vi "Get SMO Database Paths.vi"(5 "getAll Cluster":variant, 7 "Paths":string="llab_038:d000(TEST_TABLE--Temperature(Kelvin))\nllab_038:d002(TEST_TABLE--voltage 2(volts))\nllab_038:b000(TEST_TABLE--ON?())\nllab_038:v001(TEST_TABLE--sample())", 8 "error in (no error)":errorcluster, 11 "Instrument.AFM_DLog in":refnum<class "Instrument.AFM_DLog.lvclass">) -> (0 "error out":errorcluster, 2 "Paths":string, 3 "Instrument.AFM_DLog out":refnum<class "Instrument.AFM_DLog.lvclass">)   [LabVIEW 2019, in "Instrument.AFM_DLog.lvclass"]
uses:
  Instrument.AFM_DLog.lvclass
  Typedefs/Instrument.AFM_DLog.getAll--Cluster.ctl
  Typedefs/Instrument.AFM_DLog.getAll_Asylum--Cluster.ctl
  <userlib>/LevyLab/LV-Data/LV-Data.PG/API/Write Variable (one-row).vi
  <userlib>/LevyLab/Instrument Framework/Instrument Types/SCPI/Instrument.SCPI.lvclass
  <userlib>/LevyLab/LV-Data/LV-Data.PG/LV-Data.PGSQL.lvclass
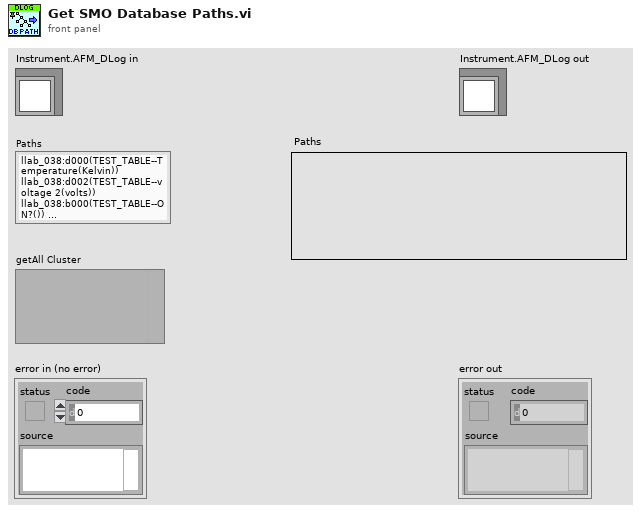
[diagram p1: front panel]
types:
  T1 = typedef "Instrument.AFM_DLog.lvclass/Instrument.AFM_DLog.getAll--Cluster.ctl" = cluster{"Name":string, "Time":string, "X":dbl, "Y":dbl, "Speed":dbl, "Voltage":dbl, "Set Resistance":string}
  T2 = typedef "Instrument.AFM_DLog.lvclass/Instrument.AFM_DLog.getAll_Asylum--Cluster.ctl" = cluster{"Time":string, "Move Setpoint":dbl, "Amplifier":dbl, "Writing Setpoint":dbl, "Interpolation":dbl}
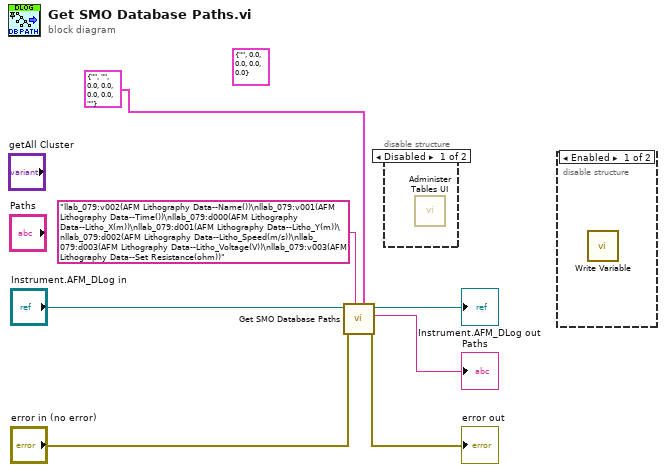
[diagram p0: block diagram]
diagram:
  (unwired) T2 {"Time"="", "Move Setpoint"=0.0, "Amplifier"=0.0, "Writing Setpoint"=0.0, "Interpolation"=0.0} ("getAll")
  n1 = call-parent "Get SMO Database Paths.vi"("getAll Cluster"=T1 {"Name"="", "Time"="", "X"=0.0, "Y"=0.0, "Speed"=0.0, "Voltage"=0.0, "Set Resistance"=""} ("getAll"), "Default Paths"="llab_079:v002(AFM Lithography Data--Name())\nllab_079:v001(AFM Lithography Data--Time())\nllab_079:d000(AFM Lithography Data--Litho_X(m))\nllab_079:d001(AFM Lithography Data--Litho_Y(m))\nllab_079:d002(AFM Lithography Data--Litho_Speed(m/s))\nllab_079:d003(AFM Lithography Data--Litho_Voltage(V))\nllab_079:v003(AFM Lithography Data--Set Resistance(ohm))" ("Paths"), "error in (no error)"="error in (no error)", "Instrument in"="Instrument.AFM_DLog in") -> ("error out"=→"error out":errorcluster, "Paths"=→"Paths":string, "Instrument out"=→"Instrument.AFM_DLog out":refnum<class "Instrument.AFM_DLog.lvclass">)  [unwired: 5 in]
  n2 = disable-structure shown="Disabled" {
    frame Disabled {
      n3 = call <userlib>:"Administer Tables UI.vi"() -> ()  [unwired: 12 in]
    }
    frame Enabled {
    }
  }
  n4 = disable-structure shown="Enabled" {
    frame Enabled {
      n5 = call-poly <userlib>:"Write Variable.vi"() -> ()  [unwired: 8 in, 4 out]
    }
    frame Disabled {
    }
  }
